vi "get config and information of the device.vi"(8 "error in":errorcluster, 11 "Dev Addr":u8=250) -> (0 "error out":errorcluster, 1 "Actual address":u8, 2 "disabled items for Channel selector":i32[](array[numeric]), 3 "Status of all channels":string[](array[string]), 4 "compensated temperature range":string, 5 "Serial number":i32, 6 "compensated pressure range":string, 7 "SW-Version":string)   [LabVIEW 2014]
uses:
  K_S30c_dll.lvlib
panel:
  out "CfgDAC":u8 format="%.0b"
  out "CfgCH0":u8
  out "Status":u8 format="%.0b"
  out "active channels":u8 format="%.0b"
  in  "Channel":enum16{"CH0", "P1", "P2", "T", "TOB1", "TOB2"}(ring)
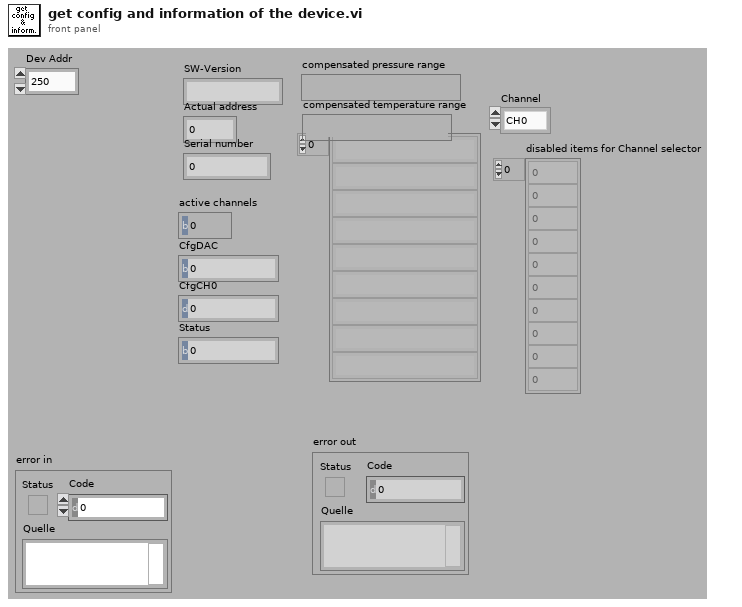
[diagram p1: front panel]
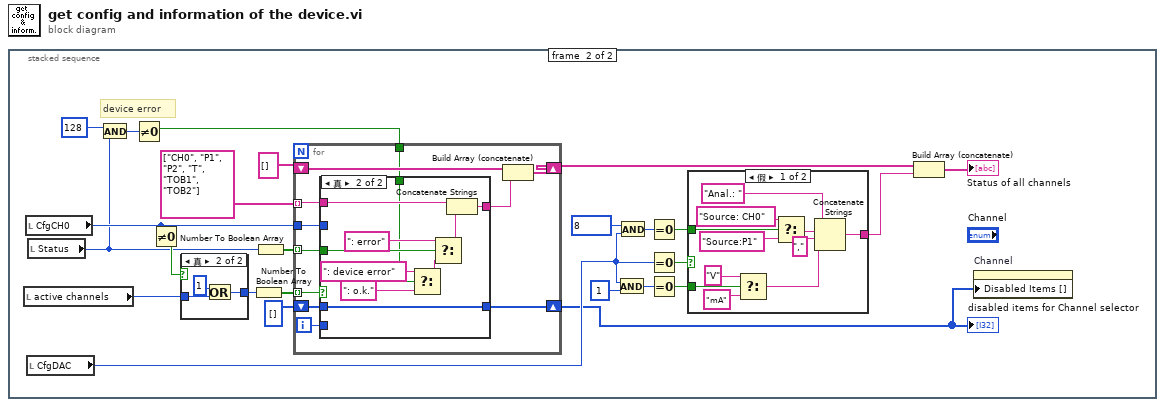
[diagram p0: block diagram]
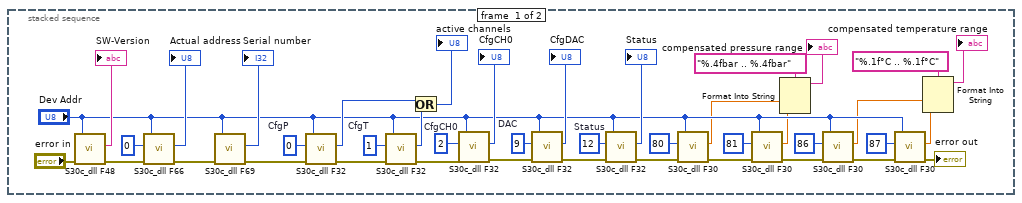
[diagram p2: hidden frame]
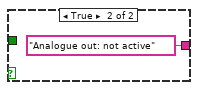
[diagram p3: hidden frame]
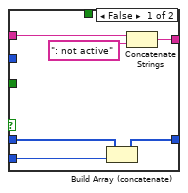
[diagram p5: hidden frame]
diagram:
  n1 = stacked-sequence {
    frame #0 {
      w28 = u8 12  # Status
      w27 = u8 9  # DAC
      w26 = u8 2  # CfgCH0
      w33 = u8 1  # CfgT
      w34 = u8 0  # CfgP
      n2 = call "S30c_dll F48.vi"("error in"="error in", "Dev Addr"="Dev Addr") -> ("error out"=w41:errorcluster, "SW-Version"=→"SW-Version":string)  [unwired: 3 in, 1 out]
      n3 = call "S30c_dll F66.vi"("error in"=w41, "New address"=u8 0, "Dev Addr"="Dev Addr") -> ("error out"=w37:errorcluster, "Actual address"=→"Actual address":u8)  [unwired: 3 in]
      n4 = call "S30c_dll F69.vi"("error in"=w37, "Dev Addr"="Dev Addr") -> ("error out"=w36:errorcluster, "Serial number"=→"Serial number":i32)  [unwired: 4 in]
      n5 = call "S30c_dll F32.vi"("error in"=w36, "Nr."=w34, "Dev Addr"="Dev Addr") -> ("error out"=w32:errorcluster, "Config Byte"=w22:u8)  [unwired: 3 in]
      n6 = call "S30c_dll F32.vi"("error in"=w32, "Nr."=w33, "Dev Addr"="Dev Addr") -> ("error out"=w31:errorcluster, "Config Byte"=w21:u8)  [unwired: 3 in]
      n7 = Or(x=w22, y=w21) -> (x .or. y?=→"active channels":u8)
      n8 = call "S30c_dll F32.vi"("error in"=w31, "Nr."=w26, "Dev Addr"="Dev Addr") -> ("error out"=w30:errorcluster, "Config Byte"=→"CfgCH0":u8)  [unwired: 3 in]
      n9 = call "S30c_dll F32.vi"("error in"=w30, "Nr."=w27, "Dev Addr"="Dev Addr") -> ("error out"=w29:errorcluster, "Config Byte"=→"CfgDAC":u8)  [unwired: 3 in]
      n10 = call "S30c_dll F32.vi"("error in"=w29, "Nr."=w28, "Dev Addr"="Dev Addr") -> ("error out"=w19:errorcluster, "Config Byte"=→"Status":u8)  [unwired: 3 in]
      n11 = call "S30c_dll F30.vi"("error in"=w19, "Nr."=u8 80, "Dev Addr"="Dev Addr") -> ("error out"=w13:errorcluster, "Coefficient"=w5:sgl)  [unwired: 3 in]
      n12 = call "S30c_dll F30.vi"("error in"=w13, "Nr."=u8 81, "Dev Addr"="Dev Addr") -> ("error out"=w12:errorcluster, "Coefficient"=w6:sgl)  [unwired: 3 in]
      n13 = Format Into String(format string="%.4fbar .. %.4fbar" ("Format-String"), w5, w6) -> (resulting string=→"compensated pressure range":string)  [unwired: 2 in, 1 out]
      n14 = call "S30c_dll F30.vi"("error in"=w12, "Nr."=u8 86, "Dev Addr"="Dev Addr") -> ("error out"=w11:errorcluster, "Coefficient"=w7:sgl)  [unwired: 3 in]
      n15 = call "S30c_dll F30.vi"("error in"=w11, "Nr."=u8 87 ("Tmax"), "Dev Addr"="Dev Addr") -> ("error out"=→"error out":errorcluster, "Coefficient"=w8:sgl)  [unwired: 3 in]
      n16 = Format Into String(format string="%.1f°C .. %.1f°C" ("Format-String"), w7, w8) -> (resulting string=→"compensated temperature range":string)  [unwired: 2 in, 1 out]
    }
    frame #1 {
      # "device error"
      n17 = local read "active channels"() -> (w53:u8)
      n18 = local read "CfgCH0"() -> (w52:u8)
      n19 = local read "CfgDAC"() -> (w60:u8)
      n20 = local read "Status"() -> (w46:u8)
      n21 = And(x=u8 128, y=w46) -> (x .and. y?=w44:u8)
      n22 = Not Equal To 0?(x=w44) -> (x != 0?=w42:bool)
      n23 = Not Equal To 0?(x=w52) -> (x != 0?=w54:bool)
      n24 = case shown="真" w54 {
        tunnel: w53 -> [w79 w82]
        tunnel: [w79 w80] -> w55
        frame False {
        }
        frame True {
          n25 = Or(x=u8 1, y=w82) -> (x .or. y?=w80:u8)
        }
      }
      n26 = Number To Boolean Array(number=w55) -> (Boolean array=w51:bool[])
      n27 = Number To Boolean Array(number=w46) -> (Boolean array=w50:bool[])
      n28 = for {
        tunnel: w50 -> [w89] mode=indexing
        shift-right: [w90] -> w64
        shift-left: string[] [] -> [w91]
        tunnel: string[] ["CH0", "P1", "P2", "T", "TOB1", "TOB2"] ("Strings []") -> [w93] mode=indexing
        tunnel: w51 -> [w88] mode=indexing
        tunnel: w52 -> [w86]
        shift-right: [w85] -> w47
        shift-left: i32[] [] -> [w84]
        tunnel: w42 -> [w83]
        i -> [w87]
        n29 = case shown="真" w88 {
          tunnel: w93 -> [w99 w109]
          tunnel: [w98 w108] -> w92
          tunnel: w89 -> [_ w106]
          tunnel: w87 -> [w96 _]
          tunnel: w86 -> [_ _]
          tunnel: [w95 w104] -> w85
          tunnel: w84 -> [w94 w104]
          tunnel: w83 -> [_ w100]
          frame False {
            n30 = Build Array (concatenate)(w94, w96) -> (w95:i32[])
            n31 = Concatenate Strings(w99, ": not active" ("String")) -> (w98:string)
          }
          frame True {
            n32 = Select(t=": device error", s=w100, f=": o.k.") -> (s? t:f=w102:string)
            n33 = Select(t=": error" ("String"), s=w106, f=w102) -> (s? t:f=w105:string)
            n34 = Concatenate Strings(w109, w105) -> (w108:string)
          }
        }
        n35 = Build Array (concatenate)(w91, w92) -> (w90:string[])
      }
      "disabled items for Channel selector" <- w47
      n36 = And(x=w60, y=u8 1) -> (x .and. y?=w58:u8)
      n37 = And(x=u8 8 ("y"), y=w60) -> (x .and. y?=w62:u8)
      n38 = Equal To 0?(x=w62) -> (x = 0?=w63:bool)
      n39 = Equal To 0?(x=w60) -> (x = 0?=w56:bool)
      n40 = Equal To 0?(x=w58) -> (x = 0?=w59:bool)
      n41 = case shown="假" w56 {
        tunnel: w59 -> [w77 _]
        tunnel: w63 -> [w72 _]
        tunnel: [w67 "Analogue out: not active"] -> w65
        frame False {
          n42 = Select(t="V", s=w77, f="mA") -> (s? t:f=w68:string)
          n43 = Select(t="Source: CH0", s=w72, f="Source:P1") -> (s? t:f=w70:string)
          n44 = Concatenate Strings("Anal.: ", w70, "," ("String"), w68) -> (w67:string)
        }
        frame True {
        }
      }
      n45 = Build Array (concatenate)(w64, w65) -> (→"Status of all channels":string[])
      n46 = property on="Channel" class="Enum (严格)"("Disabled Items []"=w47) -> ()  [unwired: 2 in, 2 out]
    }
  }
